vi "Release-motors.vi"(8 "error in (no error)":errorcluster, 11 "Object ref in":T1) -> (0 "error out":errorcluster, 3 "Object ref out":T1)   [LabVIEW 2013, in "PowderDeposition.lvlib" / "PD-Main.lvclass"]
uses:
  PD-Main.lvclass
  Object-reference.ctl
  PD-Main.lvclass/PD-Main.ctl
  Read Motor assembly.vi
  Assembly/Motor-assembly.lvclass
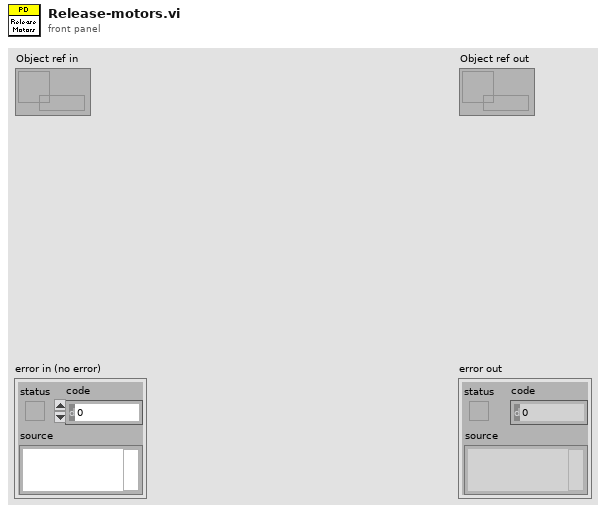
[diagram p1: front panel]
types:
  T1 = typedef "PowderDeposition.lvlib/PD-Main.lvclass/Object-reference.ctl" = refnum<data-value>
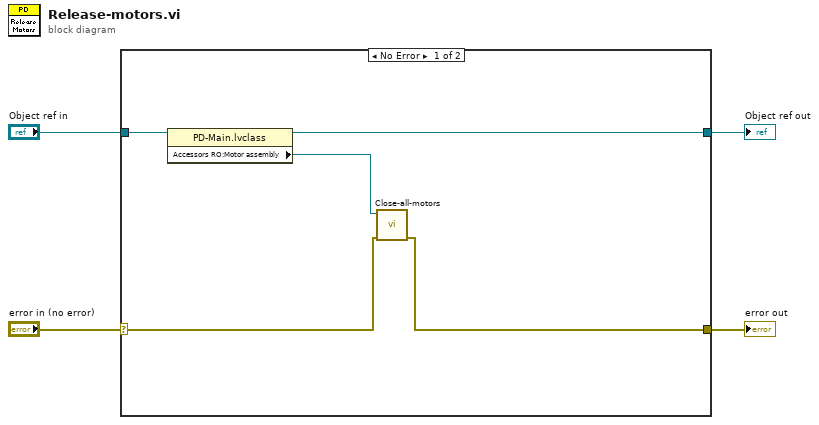
[diagram p0: block diagram]
diagram:
  n1 = case shown="No Error" "error in (no error)" {
    selector: "error in (no error)" -> [w7 w11]
    tunnel: [w6 w11] -> w3
    tunnel: [w8 w10] -> w1
    tunnel: "Object ref in" -> [w9 w10]
    frame No Error {
      n2 = property class="PD-Main.lvclass"(reference=w9) -> (reference out=w8:T1, "Accessors RO:Motor assembly"=w5:refnum<class "Motor-assembly.lvclass">)  [unwired: 1 in, 1 out]
      n3 = call "Close-all-motors.vi"("error in (no error)"=w7, "Available motors in"=w5) -> ("error out"=w6:errorcluster)  [unwired: 8 in, 1 out]
    }
    frame Error {
    }
  }
  "error out" <- w3
  "Object ref out" <- w1
